vi "send_HVBatteryStatus.vi"(4 "Counter":i32, 5 "200/freq":i32=1, 6 "Active":bool, 7 "CAN ID":u32=532 format="%x", 8 "Message":T2={"Before [V]"=600.0, "After [V]"=600.0, "Current [A]"=0.0, "SoC [mAh]"=0.0} {"SoC [mAh]" scale=0.0..65000.0; "Current [A]" scale=0.0..80.0; "After [V]" scale=0.0..700.0; "Before [V]" scale=0.0..700.0}, 11 "CAN frame":T1[](array[typedef]) {"Data" format="%.0x"; "ArbitrationId" format="%.0x"; "Timestamp" format="%<%I:%M:%S%3u %p\n%m/%d/%Y>T"}) -> (3 "CAN frame out":T1[](array[typedef]) {"Data" format="%.0x"; "ArbitrationId" format="%.0x"; "Timestamp" format="%<%I:%M:%S%3u %p\n%m/%d/%Y>T"})   [LabVIEW 2017]
uses:
  <vilib>/nican/nican.llb/CanFrameTimed.ctl
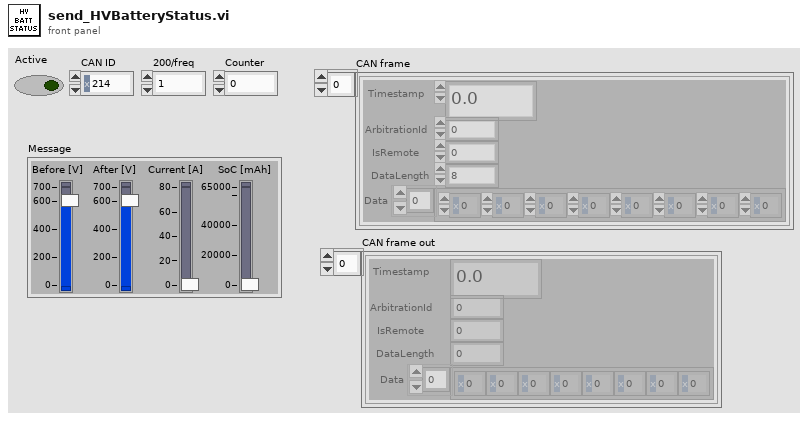
[diagram p1: front panel]
types:
  T1 = typedef "CanFrameTimed.ctl" = cluster{"Timestamp":dbl, "ArbitrationId":u32, "IsRemote":u8, "DataLength":u8, "Data":u8[]}
  T2 = cluster{"Before [V]":dbl, "After [V]":dbl, "Current [A]":dbl, "SoC [mAh]":dbl}
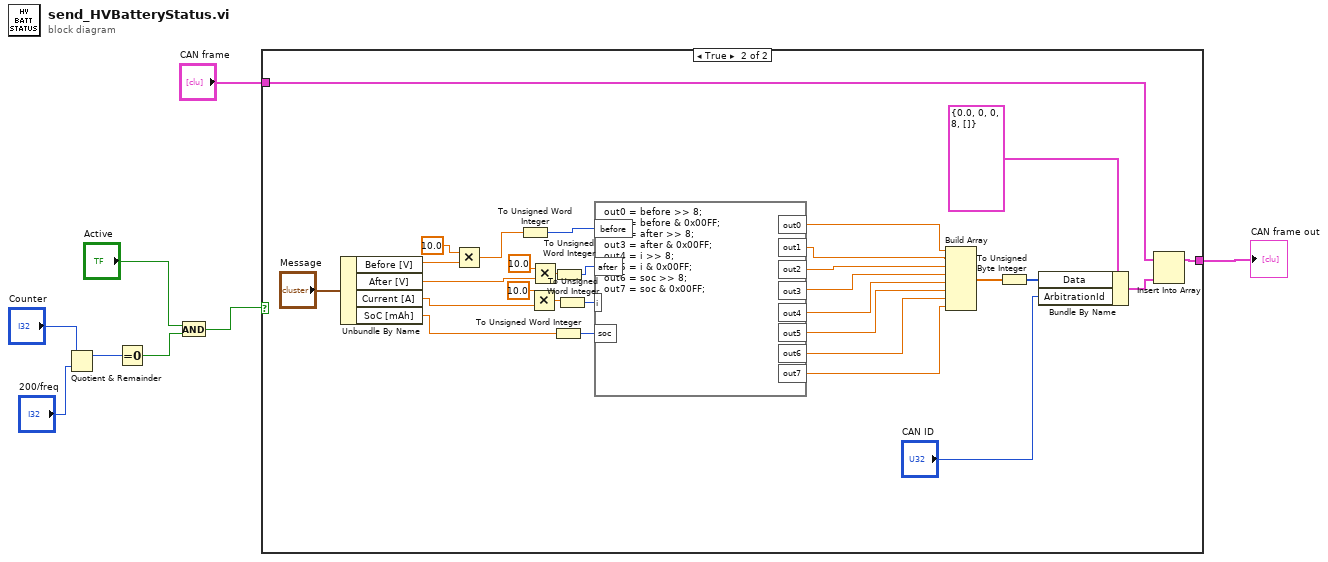
[diagram p0: block diagram]
diagram:
  n1 = Quotient & Remainder(x="Counter", y="200/freq") -> (x-y*floor(x/y)=w5:i32)  [unwired: 1 out]
  n2 = Equal To 0?(x=w5) -> (x = 0?=w3:bool)
  n3 = And(x="Active", y=w3) -> (x .and. y?=w2:bool)
  n4 = case shown="True" w2 {
    tunnel: "CAN frame" -> [w9 w31]
    tunnel: [w9 w29] -> w7
    frame False {
    }
    frame True {
      n5 = Unbundle By Name("Message") -> ("Before [V]"=w26:dbl, "After [V]"=w22:dbl, "Current [A]"=w17:dbl, "SoC [mAh]"=w15:dbl)
      n6 = Multiply(x=10.0, y=w26) -> (x*y=w25:dbl)
      n7 = To Unsigned Word Integer(number=w25) -> (unsigned 16bit integer=w27:u16)
      n8 = Multiply(x=10.0, y=w17) -> (x*y=w19:dbl)
      n9 = Multiply(x=10.0, y=w22) -> (x*y=w21:dbl)
      n10 = To Unsigned Word Integer(number=w15) -> (unsigned 16bit integer=w16:u16)
      n11 = To Unsigned Word Integer(number=w21) -> (unsigned 16bit integer=w39:u16)
      n12 = To Unsigned Word Integer(number=w19) -> (unsigned 16bit integer=w18:u16)
      n13 = formula code="out0 = before >> 8;\nout1 = before & 0x00FF;\nout2 = after >> 8;\nout3 = after & 0x00FF;\nout4 = i >> 8;\nout5 = i & 0x00FF;\nout6 = soc >> 8;\nout7 = soc & 0x00FF;"("after"=w39, "before"=w27, "i"=w18, "soc"=w16) -> ("out1"=w38:dbl, "out2"=w37:dbl, "out3"=w36:dbl, "out0"=w11:dbl, "out4"=w35:dbl, "out5"=w14:dbl, "out6"=w12:dbl, "out7"=w13:dbl)
      n14 = Build Array(w11, w38, w37, w36, w35, w14, w12, w13) -> (w34:dbl[])
      n15 = To Unsigned Byte Integer(number=w34) -> (unsigned 8bit integer=w33:u8[])
      n16 = Bundle By Name(cluster=T1 {"Timestamp"=0.0, "ArbitrationId"=0, "IsRemote"=0, "DataLength"=8, "Data"=[]} ("CAN frame"), "Data"=w33, "ArbitrationId"="CAN ID") -> (w30:T1)
      n17 = Insert Into Array(array=w31, new element=w30) -> (w29:T1[])  [unwired: 1 in]
    }
  }
  "CAN frame out" <- w7
